vi "Send Multipliers Notifier.vi"(4 "Multipliers":dbl[](array[slide])=[0.9999999999999999, 0.9999999999999999, 1.0204081632653061, 0.9999999999999999, 0.9999999999999999, 0.9999999999999999, 1.0204081632653061, 0.9999999999999999, 0.9999999999999999, 0.9999999999999999] min=0.0 max=2.0 scale=0.0..2.0) -> ()   [LabVIEW 2015]
panel:
  out "x > 0?":bool
  out "error out":errorcluster
  in  "error in (no error)":errorcluster
  # "1"
  # "2"
  # "3"
  # "4"
  # "5"
  # "6"
  # "7"
  # "8"
  # "9"
  # "10"
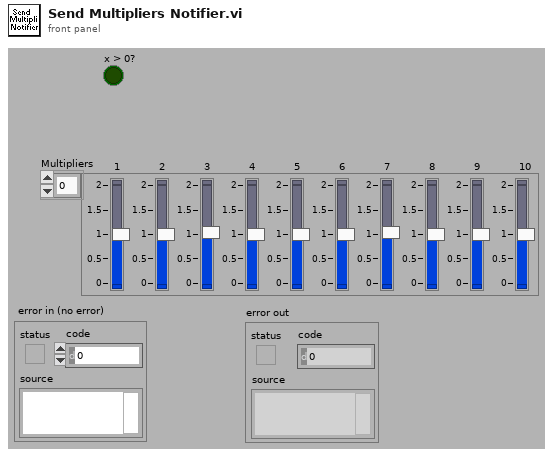
[diagram p1: front panel]
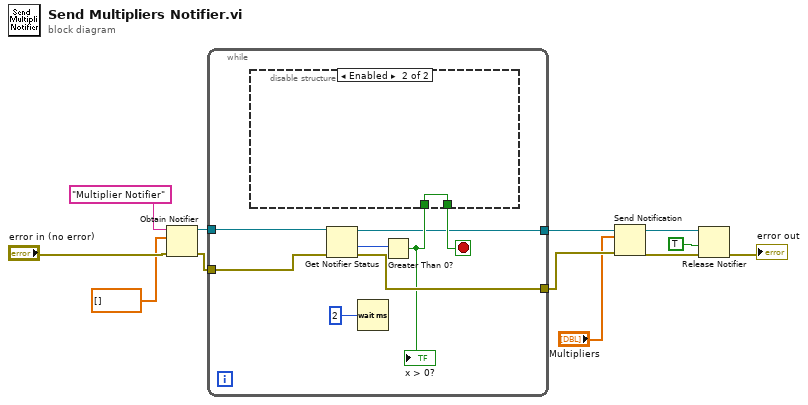
[diagram p0: block diagram]
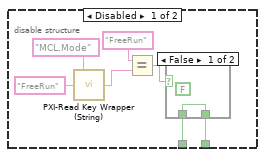
[diagram p2: hidden frame]
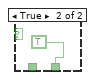
[diagram p3: hidden frame]
diagram:
  n1 = Obtain Notifier(name (unnamed)="Multiplier Notifier", notification data type=dbl[] [], error in (no error)="error in (no error)") -> (notifier out=w3:refnum<notifier>, error out=w5:errorcluster)  [unwired: 1 in, 1 out]
  n2 = while {
    tunnel: w5 -> [w19]
    tunnel: [w17] -> w4
    tunnel: w3 -> [w14]
    tunnel: [w13] -> w2
    stop <- w15 stop-if-true
    n3 = Get Notifier Status(notifier=w14, error in (no error)=w19) -> (notifier out=w13:refnum<notifier>, # waiting=w18:i32, error out=w17:errorcluster)  [unwired: 2 out]
    n4 = Wait (ms)(milliseconds to wait=2) -> ()  [unwired: 1 out]
    n5 = Greater Than 0?(x=w18) -> (x > 0?=w16:bool)
    "x > 0?" <- w16
    n6 = disable-structure shown="Enabled" {
      disable-tunnel: w16 -> [w22 w30]
      disable-tunnel: [w21 w30] -> w15
      frame Disabled {
        n7 = call "PXI-Read Key Wrapper (String).vi"("key"="MCL.Mode", "default value"="FreeRun") -> ("value"=w25:string)  [unwired: 11 in, 2 out]
        n8 = Equal?(x="FreeRun" ("default value"), y=w25) -> (x = y?=w23:bool)
        n9 = case shown="False" w23 {
          tunnel: w22 -> [w28 _]
          tunnel: [w28 TRUE] -> w21
          frame False {
            (unwired) FALSE
          }
          frame True {
          }
        }
      }
      frame Enabled {
      }
    }
  }
  n10 = Send Notification(notification="Multipliers", notifier=w2, error in (no error)=w4) -> (notifier out=w9:refnum<notifier>, error out=w8:errorcluster)
  n11 = Release Notifier(notifier=w9, force destroy? (F)=TRUE, error in (no error)=w8) -> (error out=→"error out":errorcluster)  [unwired: 2 out]
